vi "Pre Launch Init.vi"(11 "Map Model in":refnum<class "Map Model.lvclass">) -> (0 "error out":errorcluster, 3 "Map Model out":refnum<class "Map Model.lvclass">)   [LabVIEW 2020, in "Map Model.lvlib" / "Map Model.lvclass"]
doc: "(<B>Filename</B>: Actor Framework.lvlib:Actor.lvclass:Pre Launch Init.vi)\n\nDefines behavior that occurs after the Launch Nested Actor method is invoked but before the actor's Actor Core method begins running.\n\nBy default, this method does nothing. A descendant class may override it to define behavior."
uses:
  Map Model.lvclass
  Tools/Pan/Pan.lvclass
  E:/Project/Labview-Projects/Completed projects/Map Editor/Models/Map Model/Tools/Tool/Tool.lvclass
  Stack/Stack.lvclass
  Map Model.lvclass/Map Model.ctl
  <vilib>/ActorFramework/Actor/Actor.lvclass
panel:
  # "NOTICE -- YOU MUST LEAVE THIS NOTICE IN PLACE.\n\nCopyright (c) 2017, LIANG LIU Shawn.Liu.cn@gmail.com\nAll rights reserved.\n\nRedistribution and use in source and binary forms, with or without modification, are permitted provided that the following conditions are met:\n-Redistributions of source code must retain the above copyright notice, this list of conditions and the following disclaimer.\n-Redistributions in binary form must reproduce the above copyright notice, this list of conditions and the following disclaimer in the documentation and/or other materials provided with the distribution.\n-Neither the name of the eLp nor the names of its contributors may be used to endorse or promote products derived from this software without specific prior written permission.\n\nTHIS SOFTWARE IS PROVIDED BY THE COPYRIGHT HOLDERS AND CONTRIBUTORS \"AS IS\" AND ANY EXPRESS OR IMPLIED WARRANTIES, INCLUDING, BUT NOT LIMITED TO, THE IMPLIED WARRANTIES OF MERCHANTABILITY AND FITNESS FOR A PARTICULAR PURPOSE ARE DISCLAIMED. IN NO EVENT SHALL THE COPYRIGHT HOLDER OR CONTRIBUTORS BE LIABLE FOR ANY DIRECT, INDIRECT, INCIDENTAL, SPECIAL, EXEMPLARY, OR CONSEQUENTIAL DAMAGES (INCLUDING, BUT NOT LIMITED TO, PROCUREMENT OF SUBSTITUTE GOODS OR SERVICES; LOSS OF USE, DATA, OR PROFITS; OR BUSINESS INTERRUPTION) HOWEVER CAUSED AND ON ANY THEORY OF LIABILITY, WHETHER IN CONTRACT, STRICT LIABILITY, OR TORT (INCLUDING NEGLIGENCE OR OTHERWISE) ARISING IN ANY WAY OUT OF THE USE OF THIS SOFTWARE, EVEN IF ADVISED OF THE POSSIBILITY OF SUCH DAMAGE."
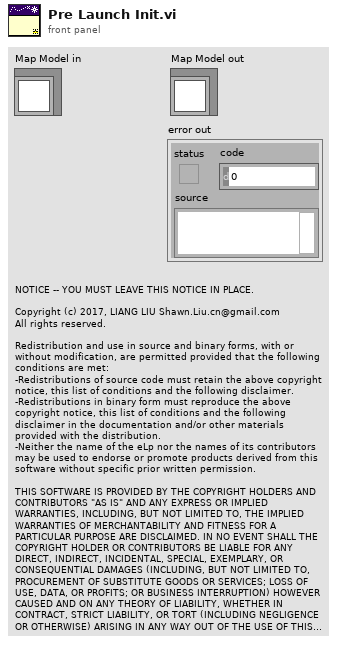
[diagram p1: front panel]
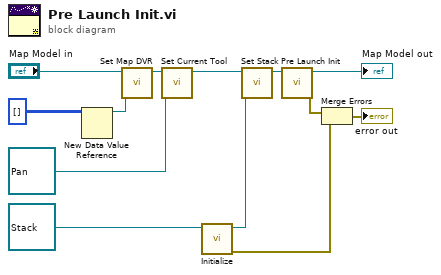
[diagram p0: block diagram]
diagram:
  n1 = New Data Value Reference(data value=u8[][] []) -> (data value reference=w10:refnum<data-value>)  [unwired: 1 in, 1 out]
  n2 = call "Set Map DVR.vi"("Map DVR"=w10, "Map Model in"="Map Model in") -> ("Map Model out"=w1:refnum<class "Map Model.lvclass">)  [unwired: 9 in]
  n3 = call "Set Current Tool.vi"("Current Tool"=refnum<class "Pan.lvclass"> refnum ("Map Model.lvlib:Pan.lvclass"), "Map Model in"=w1) -> ("Map Model out"=w3:refnum<class "Map Model.lvclass">)  [unwired: 9 in]
  n4 = call "Initialize.vi"("Stack in"=refnum<class "Stack.lvclass"> refnum ("Map Model.lvlib:Stack.lvclass")) -> ("error out"=w4:errorcluster, "Stack out"=w6:refnum<class "Stack.lvclass">)  [unwired: 9 in]
  n5 = call "Set Stack.vi"("Stack"=w6, "Map Model in"=w3) -> ("Map Model out"=w8:refnum<class "Map Model.lvclass">)  [unwired: 9 in]
  n6 = call-parent "Pre Launch Init.vi"("Actor in"=w8) -> ("error out"=w11:errorcluster, "Actor out"=→"Map Model out":refnum<class "Map Model.lvclass">)  [unwired: 9 in]
  n7 = Merge Errors(w11, w4) -> (→"error out":errorcluster)
